vi "DS_Mode_Simulation_Global.vi"(0 "menu":enum16{"set", "get"}(ring)=enum."get", 7 "simulated? in":bool, 11 "error in (no error)":errorcluster) -> (8 "simulated? out":bool, 15 "error out":errorcluster)   [LabVIEW 2017]
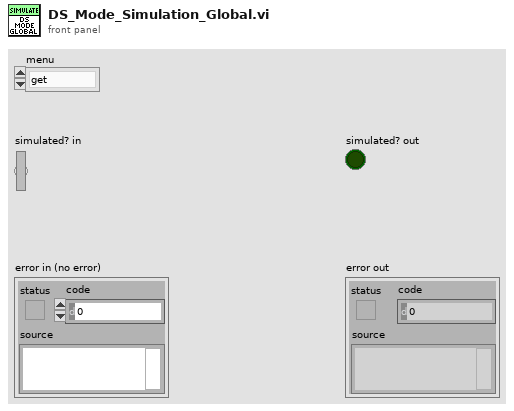
[diagram p1: front panel]
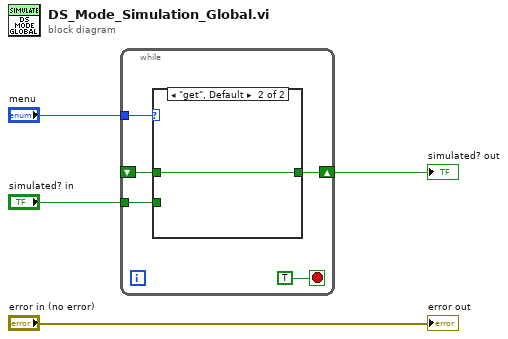
[diagram p0: block diagram]
diagram:
  n1 = while {
    tunnel: "menu" -> [w8]
    shift-right: [w6] -> w1
    shift-left: _ -> [w7]
    tunnel: "simulated? in" -> [w5]
    stop <- TRUE stop-if-true
    n2 = case shown="\"get\", Default" w8 {
      tunnel: w7 -> [_ w11]
      tunnel: [w10 w11] -> w6
      tunnel: w5 -> [w10 _]
      frame "set" {
      }
      frame "get", Default {
      }
    }
  }
  "simulated? out" <- w1
  "error out" <- "error in (no error)"
